vi "Format Fit Output.vi"(5 "Fit Model":T4, 7 "f(x,a)":T1, 8 "Error In":errorcluster, 9 "Fit Results":T2, 10 "Additional Data":variant, 11 "Data in":T3) -> (0 "Error Out":errorcluster, 1 "Fit Parameters Uncertainties Cluster":variant, 3 "Fit Parameters Cluster":variant)   [LabVIEW 2021, in "Fits.lvlib"]
uses:
  Fits.lvlib
  Fit Models.ctl
  <vilib>/gmath/NumericalOptimization/LM model function reference.ctl
  <vilib>/Utility/error.llb/DialogType.ctl
  Gaussian/Gaussian Fit Results v2.ctl
  Asymmetric Gaussian/Asymmetric Gaussian Fit Results v2.ctl
  Lorentzian/Lorentzian Fit Results v2.ctl
  Asymmetric Lorentzian/Asymmetric Lorentzian Fit Results v2.ctl
  Gaussian-Lorentzian/Gaussian-Lorentzian Fit Results v2.ctl
  Lorentzian-Gaussian/Lorentzian-Gaussian Fit Results v2.ctl
  D-Only Fixed Parameters.ctl
  Two Connected Gaussians/Two H-Connected Gaussians Fit Parameters.ctl
  Two Connected Gaussians/Two T-Connected Gaussians Fit Parameters.ctl
  Two Connected Asymmetric Gaussians/Two H-Connected Asymmetric Gaussians Fit Parameters.ctl
  Two Connected Asymmetric Gaussians/Two T-Connected Asymmetric Gaussians Fit Parameters.ctl
  Single Exponential/Single Exponential Fit Parameters v2.ctl
  Power Law/Power Law Fit Parameters.ctl
  IRF(X)PSED/IRF(X)PSED Fit Parameters.ctl
  IRF(X)PSED/IRF(X)PSED Fixed Parameters v3.ctl
  IRF(X)PSED/IRF(X)PSED Extraction Options.ctl
  IRF(X)PSED/Fourier Series Smoothing Option.ctl
  IRF(X)PSED/Fourier Series Truncation.ctl
  IRF(X)PSED/IRF Extraction Method.ctl
  Double Exponential/Double Exponential Fit Parameters v2.ctl
  ACF-CCF/2D ACF/2D Gaussian ACF Fit Results.ctl
  ACF-CCF/2D ACF/2D Gaussian + Blinking ACF Fit Results.ctl
  ACF-CCF/2D ACF/2D Gaussian + Flow ACF Fit Results.ctl
  ACF-CCF/3D ACF/3D Gaussian ACF Fit Results.ctl
  ACF-CCF/3D ACF/3D Gaussian + Blinking ACF Fit Results.ctl
  ACF-CCF/2D ACF/2D Gaussian ACF & 2D Gaussian ACF + Flow Fit Results.ctl
  <vilib>/Analysis/NI_AALPro.lvlib
  <vilib>/gmath/NI_Gmath.lvlib
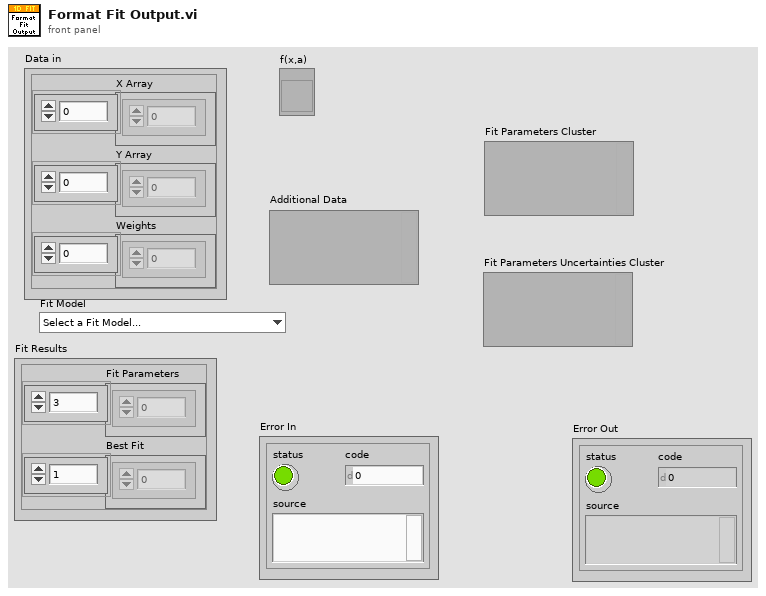
[diagram p1: front panel]
types:
  T1 = typedef "NI_Gmath.lvlib/LM model function reference.ctl" = refnum<vi>
  T2 = cluster{"Fit Parameters":dbl[], "Best Fit":dbl[]}
  T3 = cluster{"X Array":dbl[], "Y Array":dbl[], "Weights":dbl[]}
  T4 = typedef "Fits.lvlib/Fit Models.ctl" = enum16{"Select a Fit Model...", "           Single Peak", "Gaussian", "Asymmetric Gaussian", "Lorentzian", "Asymmetric Lorentzian", "Gaussian/Lorentzian", "Lorentzian/Gaussian", "           Double Peak", "Two Gaussians", "Two Asymmetric Gaussians", "Two H-Connected Gaussians", "Two T-Connected Gaussians", "Two H-Connected Asymmetric Gaussians", "Two T-Connected Asymmetric Gaussians", "           Triple Peak", "Three Gaussians", "Three Asymmetric Gaussians", "              Decays", "1-Exponential", "IRF*PSED", "2-Exponentials", "Power Law", "Power Law with Offset", "               ACF", "2D Gaussian ACF", "2D Gaussian + Blinking ACF", "2D Gaussian + Flow ACF", "3D Gaussian ACF", "3D Gaussian + Blinking ACF", "             Multiplot", "2D Gaussian ACF & 2D Gaussian + Flow ACF"}
  T5 = typedef "Fits.lvlib/D-Only Fixed Parameters.ctl" = cluster{"Fix D-only Peak Location":bool, "Peak Location":dbl, "Fix D-only Peak FWHM":bool, "Peak FWHM":dbl}
  T6 = typedef "Fits.lvlib/IRF(X)PSED Fixed Parameters v3.ctl" = cluster{"order":i32, "T":dbl, "Time Constant Array":dbl[], "{S_k, C_k, phi_k, e_k} arrays":cluster{"S_k Array":dbl[], "C_k Array":dbl[], "phi_k Array":dbl[], "e_k Array":dbl[]}, "IRF Extraction Options":T7}
  T7 = typedef "Fits.lvlib/IRF(X)PSED Extraction Options.ctl" = cluster{"Time Constant for IRF Extraction":dbl[unit], "IRF Order":i32, "Fourier Series Smoothing":T8, "Noise Threshold":dbl, "Smoothing Width":dbl, "Fourier Series Truncation":T9, "Truncation Order":i32, "Save Power Spectrum":bool, "Smoothing":bool, "Smoothing Parameter":dbl, "Smoothing Order":u32, "Method":T10}
  T8 = typedef "Fits.lvlib/Fourier Series Smoothing Option.ctl" = enum16{"None", "Lanczos Factors", "Fejer Summation"}
  T9 = typedef "Fits.lvlib/Fourier Series Truncation.ctl" = enum16{"Automatic", "Fixed"}
  T10 = typedef "Fits.lvlib/IRF Extraction Method.ctl" = enum16{"Direct", "Topless", "Toeplitz"}
  T11 = typedef "DialogType.ctl" = u16
  T12 = typedef "Fits.lvlib/Gaussian Fit Results v2.ctl" = cluster{"Amplitude":dbl, "Peak":dbl, "SDV":dbl, "FWHM":dbl, "Integral":dbl, "RMSE":dbl, "R^2":dbl}
  T13 = typedef "Fits.lvlib/Asymmetric Gaussian Fit Results v2.ctl" = cluster{"Amplitude":dbl, "Peak":dbl, "SDV-":dbl, "SDV+":dbl, "Mean":dbl, "SDV":dbl, "FWHM":dbl, "Integral":dbl, "RMSE":dbl, "R^2":dbl}
  T14 = typedef "Fits.lvlib/Lorentzian Fit Results v2.ctl" = cluster{"Amplitude":dbl, "Peak":dbl, "FWHM":dbl, "Integral":dbl, "RMSE":dbl, "R^2":dbl}
  T15 = typedef "Fits.lvlib/Asymmetric Lorentzian Fit Results v2.ctl" = cluster{"Amplitude":dbl, "Peak":dbl, "FWHM-":dbl, "FWHM+":dbl, "Integral":dbl, "RMSE":dbl, "R^2":dbl}
  T16 = typedef "Fits.lvlib/Gaussian-Lorentzian Fit Results v2.ctl" = cluster{"Amplitude":dbl, "Peak":dbl, "SDV-":dbl, "FWHM+":dbl, "Mean":dbl, "FWHM":dbl, "Integral":dbl, " RMSE":dbl, "R^2":dbl}
  T17 = typedef "Fits.lvlib/Lorentzian-Gaussian Fit Results v2.ctl" = cluster{"Amplitude":dbl, "Peak":dbl, "FWHM-":dbl, "SDV+":dbl, "Mean":dbl, "FWHM":dbl, "Integral":dbl, "RMSE":dbl, "R^2":dbl}
  T18 = typedef "Fits.lvlib/Two H-Connected Gaussians Fit Parameters.ctl" = cluster{"Gaussian Parameters":T12[], "Bridge Amplitude ":dbl}
  T19 = typedef "Fits.lvlib/Two T-Connected Gaussians Fit Parameters.ctl" = cluster{"Gaussian Parameters":T12[], "Bridge Amplitude ":dbl, "Bridge Slope":dbl}
  T20 = typedef "Fits.lvlib/Two H-Connected Asymmetric Gaussians Fit Parameters.ctl" = cluster{"Asymmetric Gaussian Parameters":T13[], "Bridge Amplitude":dbl}
  T21 = typedef "Fits.lvlib/Two T-Connected Asymmetric Gaussians Fit Parameters.ctl" = cluster{"Asymmetric Gaussian Parameters":T13[], "Bridge Amplitude":dbl, "Bridge Slope":dbl}
  T22 = typedef "Fits.lvlib/Single Exponential Fit Parameters v2.ctl" = cluster{"Amplitude":dbl, "Time Constant":dbl, "Baseline":dbl, "Mean":dbl, "SDV":dbl, "FWHM":dbl, "Integral":dbl, "MSE":dbl, "R^2":dbl}
  T23 = typedef "Fits.lvlib/Power Law Fit Parameters.ctl" = cluster{"A":dbl, "beta":dbl, "B":dbl, "Mean":dbl, "SDV":dbl, "Integral":dbl, "MSE":dbl, "R^2":dbl}
  T24 = typedef "Fits.lvlib/IRF(X)PSED Fit Parameters.ctl" = cluster{"Offset":dbl, "Amplitudes":dbl[], "Time Constants":dbl[], "Baseline":dbl, "Lifetime":dbl, "IRF order":dbl, "Period":dbl, "SDV":dbl, "FWHM":dbl, "Integral":dbl, "MSE":dbl, "R^2":dbl}
  T25 = typedef "Fits.lvlib/Double Exponential Fit Parameters v2.ctl" = cluster{"A1":dbl, "tau1":dbl, "A2":dbl, "tau2":dbl, "Baseline":dbl, "Mean":dbl, "SDV":dbl, "Integral":dbl, "MSE":dbl, "R^2":dbl}
  T26 = typedef "Fits.lvlib/2D Gaussian ACF Fit Results.ctl" = cluster{"Amplitude":dbl, "Diffusion Time":dbl, "RMSE":dbl, "R^2":dbl}
  T27 = typedef "Fits.lvlib/2D Gaussian + Blinking ACF Fit Results.ctl" = cluster{"Amplitude":dbl, "Diffusion Time":dbl, "Blinking Fraction":dbl, "Blinking Time Constant":dbl, "RMSE":dbl, "R^2":dbl}
  T28 = typedef "Fits.lvlib/2D Gaussian + Flow ACF Fit Results.ctl" = cluster{"Amplitude":dbl, "Diffusion Time":dbl, "Translation Time":dbl, "RMSE":dbl, "R^2":dbl}
  T29 = typedef "Fits.lvlib/3D Gaussian ACF Fit Results.ctl" = cluster{"Amplitude":dbl, "Diffusion Time":dbl, "Aspect Ratio":dbl, "RMSE":dbl, "R^2":dbl}
  T30 = typedef "Fits.lvlib/3D Gaussian + Blinking ACF Fit Results.ctl" = cluster{"Amplitude":dbl, "Diffusion Time":dbl, "Aspect Ratio":dbl, "Blinking Fraction":dbl, "Blinking Time Constant":dbl, "RMSE":dbl, "R^2":dbl}
  T31 = typedef "Fits.lvlib/2D Gaussian ACF & 2D Gaussian ACF + Flow Fit Results.ctl" = cluster{"Amplitude 1":dbl, "Diffusion Time":dbl, "Amplitude 2":dbl, "Translation Time":dbl, "RMSE":dbl, "R^2":dbl}
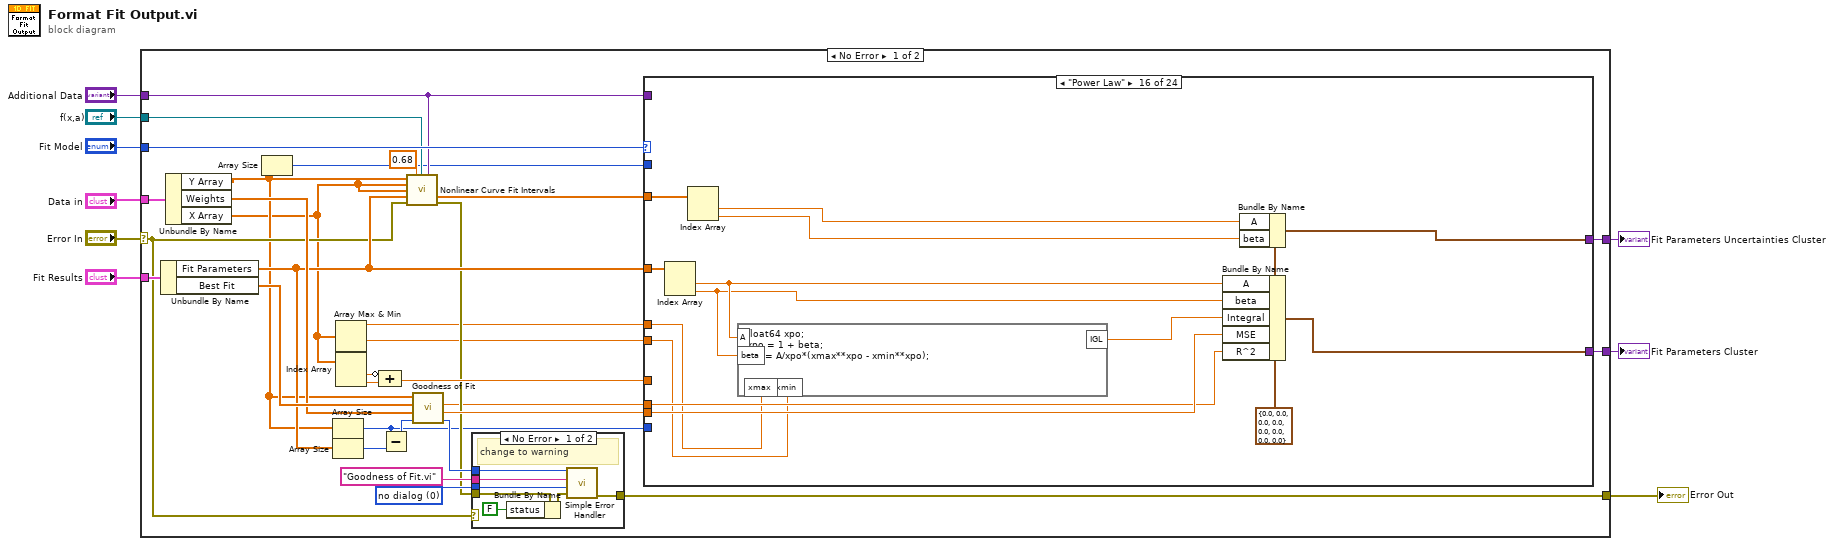
[diagram p0: block diagram]
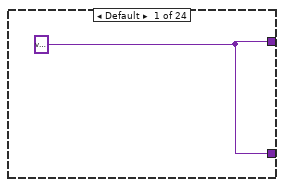
[diagram p3: hidden frame]
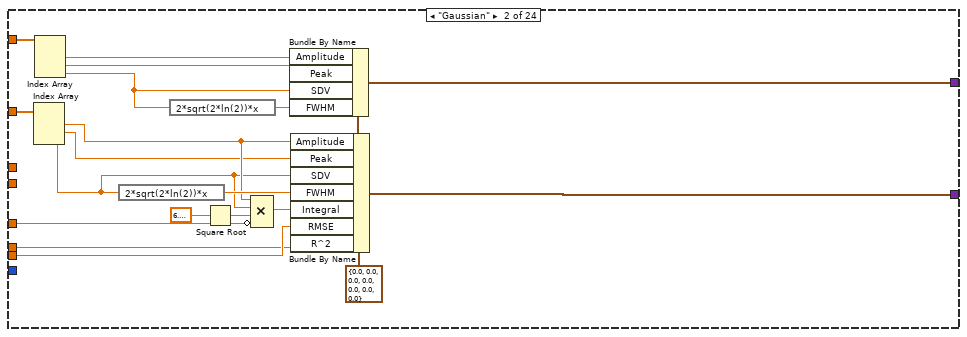
[diagram p4: hidden frame]
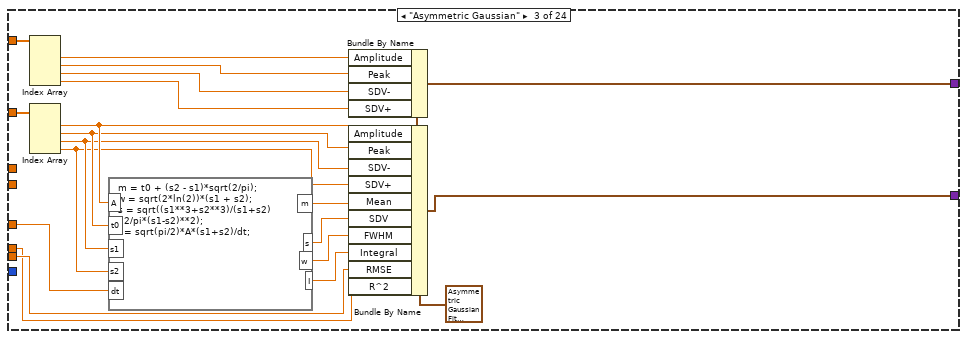
[diagram p5: hidden frame]
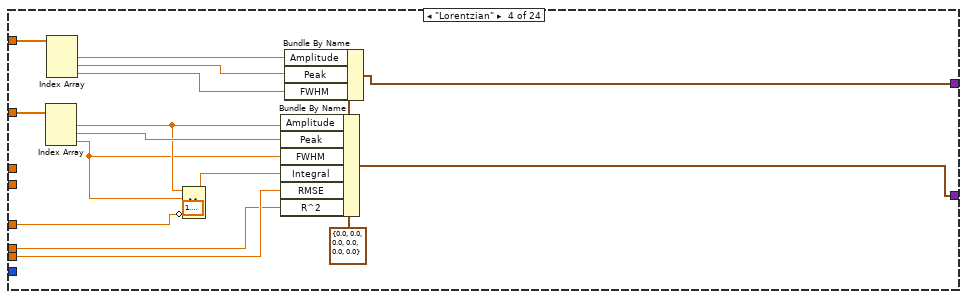
[diagram p6: hidden frame]
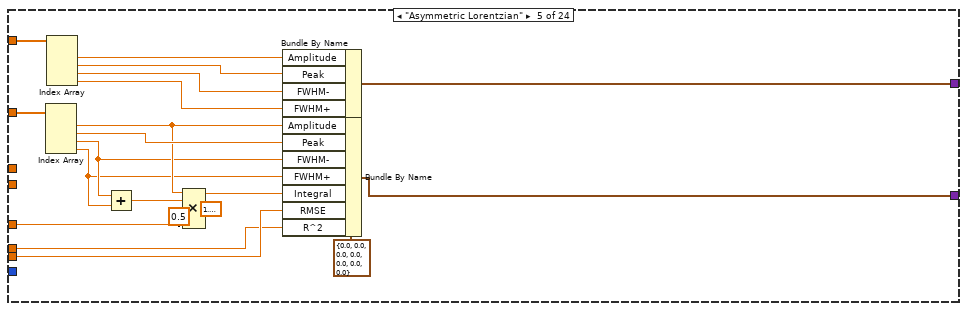
[diagram p7: hidden frame]
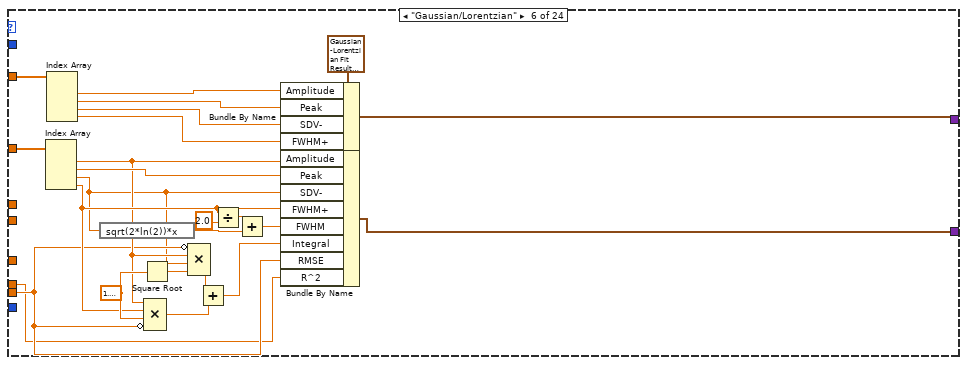
[diagram p8: hidden frame]
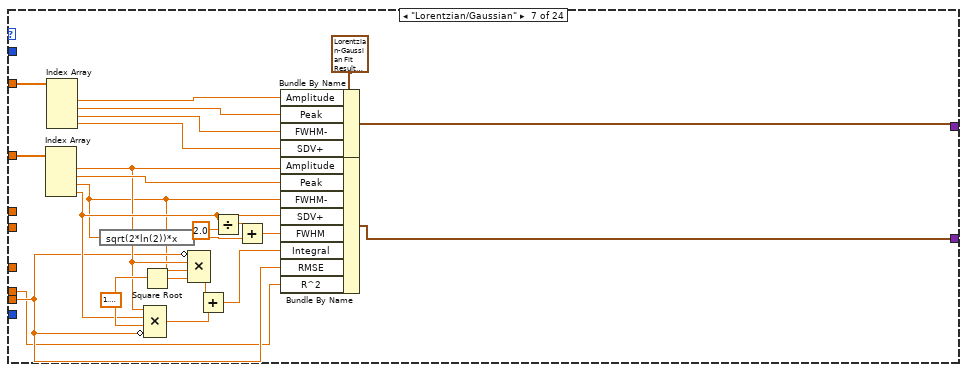
[diagram p9: hidden frame]
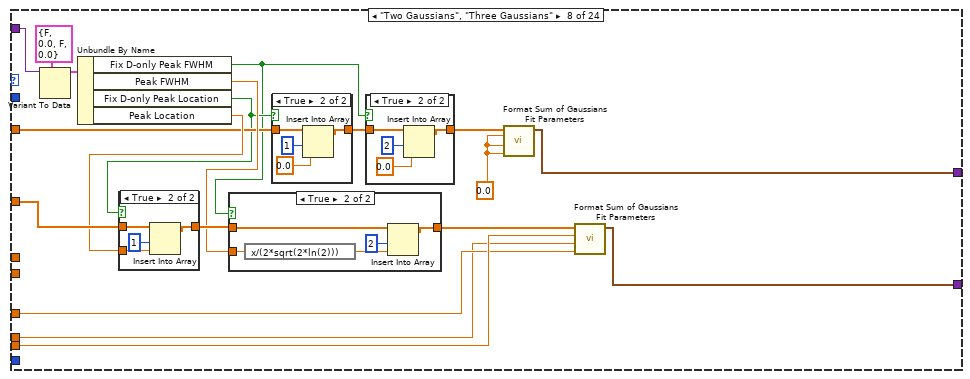
[diagram p10: hidden frame]
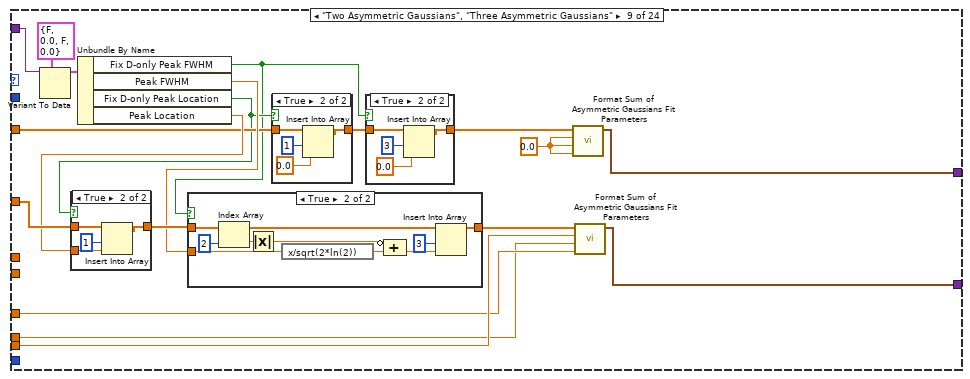
[diagram p15: hidden frame]
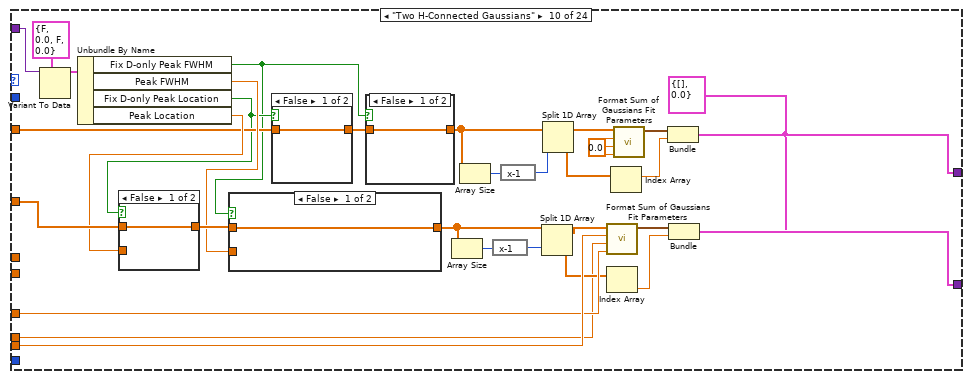
[diagram p20: hidden frame]
diagram:
  n1 = case shown="No Error" "Error In" {
    selector: "Error In" -> [w15 w667]
    tunnel: [w40 _] -> w9
    tunnel: [w39 _] -> w8
    tunnel: "Data in" -> [w32 _]
    tunnel: "Fit Results" -> [w31 _]
    tunnel: "Fit Model" -> [w29 _]
    tunnel: "f(x,a)" -> [w25 _]
    tunnel: [w20 w667] -> w2
    tunnel: "Additional Data" -> [w18 _]
    frame No Error {
      w22 = T11 0 items=["no dialog", "OK message", "continue or stop message", "OK message + warnings", "continue/stop + warnings"] ("type of dialog (OK msg:1)")
      n2 = Unbundle By Name(w31) -> ("Fit Parameters"=w27:dbl[], "Best Fit"=w30:dbl[])
      n3 = Unbundle By Name(w32) -> ("Y Array"=w14:dbl[], "Weights"=w28:dbl[], "X Array"=w12:dbl[])
      n4 = Array Size(array=w14) -> (size(s)=w13:i32)
      n5 = Array Size(array=w14) -> (size(s)=w16:i32)
      n6 = Array Size(array=w27) -> (size(s)=w35:i32)
      n7 = Array Max & Min(array=w12) -> (max value=w10:dbl, min value=w11:dbl)  [unwired: 2 out]
      n8 = Index Array(array=w12) -> (element #1=w36:dbl, element #2=w38:dbl)  [unwired: 2 in]
      n9 = Compound Arithmetic op=ADD(invert w36, w38) -> (w37:dbl)
      n10 = Subtract(x=w16, y=w35) -> (x-y=w34:i32)
      n11 = call <vilib>:"Nonlinear Curve Fit Intervals.vi"("Y"=w14, "confidence level"=0.68, "f(x,a)"=w25, "data"=w18, "X"=w12, "Weight"=w12, "best fit parameters"=w27, "error in (no error)"=w15) -> ("delta best fit parameters"=w26:dbl[], "error out"=w21:errorcluster)  [unwired: 4 in, 2 out]
      n12 = call <vilib>:"Goodness of Fit.vi"("degree of freedom"=w34, "Weight"=w28, "Best Fit"=w30, "Y"=w14) -> ("error"=w24:i32, "RMSE"=w33:dbl, "R-square"=w17:dbl)  [unwired: 4 in, 1 out]
      n13 = case shown="No Error" w15 {
        selector: w15 -> [_ w48]
        tunnel: w24 -> [w47 _]
        tunnel: "Goodness of Fit.vi" ("error source (\" \")") -> [w46 _]
        tunnel: w22 -> [w45 _]
        tunnel: w21 -> [w44 _]
        tunnel: [w43 w48] -> w20
        frame No Error {
          # "change to warning"
          n14 = Bundle By Name(cluster=w44, "status"=FALSE) -> (w42:errorcluster)
          n15 = call <vilib>:"Simple Error Handler.vi"("error code (no error:0)"=w47, "error source (\" \")"=w46, "type of dialog (OK msg:1)"=w45, "error in (no error)"=w42) -> ("error out"=w43:errorcluster)  [unwired: 1 in, 4 out]
        }
        frame Error {
        }
      }
      n16 = case shown="\"Power Law\"" w29 {
        tunnel: [w49 w56 w82 w90 w114 w142 w166 w176 w216 w274 w329 w382 w441 w489 w510 w524 w557 w576 w589 w604 w617 w632 w649 w664] -> w40
        tunnel: [w49 w55 w81 w102 w113 w141 w165 w175 w215 w275 w330 w383 w442 w488 w509 w523 w556 w568 w588 w603 w616 w631 w648 w663] -> w39
        tunnel: w37 -> [_ w59 w71 w97 w119 _ _ w178 w218 w276 w331 w384 w443 w483 _ _ w554 w574 _ _ _ _ _ _]
        tunnel: w33 -> [_ w58 w80 w103 w123 w127 w152 w179 w219 w277 w332 w385 w444 w492 w511 w525 w558 w570 w591 w606 w619 w634 w651 w666]
        tunnel: w27 -> [_ w57 w88 w104 w124 w148 w172 w188 w228 w285 w340 w393 w452 w496 w512 w526 w547 w575 w590 w605 w618 w633 w650 w665]
        tunnel: w26 -> [_ w54 w87 w95 w118 w146 w170 w184 w224 w281 w336 w389 w448 w499 w515 w529 w552 w581 w587 w602 w615 w630 w647 w662]
        tunnel: w18 -> [_ _ _ _ _ _ _ w190 w230 w287 w342 w395 w454 _ _ _ w541 _ _ _ _ _ _ _]
        tunnel: w17 -> [_ w50 w69 w89 w105 w125 w149 w174 w213 w258 w310 w365 w423 w486 w507 w522 w555 w563 w585 w600 w613 w629 w645 w660]
        tunnel: w16 -> [_ _ _ _ _ _ _ _ _ _ _ _ _ w482 _ _ w553 w561 _ _ _ _ _ _]
        tunnel: w13 -> [_ _ _ _ _ _ _ _ _ _ _ _ _ _ _ _ w532 _ _ _ _ _ _ _]
        tunnel: w11 -> [_ _ _ _ _ _ _ _ _ _ _ _ _ _ w502 w518 _ _ _ _ _ _ _ _]
        tunnel: w10 -> [_ _ _ _ _ _ _ _ _ _ _ _ _ _ w501 w517 _ _ _ _ _ _ _ _]
        frame Default {
          w49 = variant
        }
        frame "Gaussian" {
          w67 = T12 {"Amplitude"=0.0, "Peak"=0.0, "SDV"=0.0, "FWHM"=0.0, "Integral"=0.0, "RMSE"=0.0, "R^2"=0.0} ("Gaussian Fit Parameters")
          n17 = Index Array(array=w57) -> (element #1=w62:dbl, element #2=w61:dbl, element #3=w60:dbl)  [unwired: 3 in]
          n18 = Index Array(array=w54) -> (element #1=w53:dbl, element #2=w52:dbl, element #3=w51:dbl)  [unwired: 3 in]
          n19 = expression code="2*sqrt(2*ln(2))*x"(w60) -> (w66:dbl)
          n20 = expression code="2*sqrt(2*ln(2))*x"(w51) -> (w68:dbl)
          n21 = Square Root(x=6.283185307179586) -> (sqrt(x)=w64:dbl)
          n22 = Compound Arithmetic op=MULTIPLY(w62, w60, w64, invert w59) -> (w65:dbl)
          n23 = Bundle By Name(cluster=w67, "Amplitude"=w53, "Peak"=w52, "SDV"=w51, "FWHM"=w68) -> (w56:T12)
          n24 = Bundle By Name(cluster=w67, "Amplitude"=w62, "Peak"=w61, "SDV"=w60, "FWHM"=w66, "Integral"=w65, "RMSE"=w58, "R^2"=w50) -> (w55:T12)
        }
        frame "Asymmetric Gaussian" {
          w86 = T13 {"Amplitude"=0.0, "Peak"=0.0, "SDV-"=0.0, "SDV+"=0.0, "Mean"=0.0, "SDV"=0.0, "FWHM"=0.0, "Integral"=0.0, "RMSE"=0.0, "R^2"=0.0} ("Lorentz Fit Parameters")
          n25 = Index Array(array=w87) -> (element #1=w85:dbl, element #2=w84:dbl, element #3=w83:dbl, element #4=w70:dbl)  [unwired: 4 in]
          n26 = Index Array(array=w88) -> (element #1=w75:dbl, element #2=w74:dbl, element #3=w73:dbl, element #4=w72:dbl)  [unwired: 4 in]
          n27 = formula code="m = t0 + (s2 - s1)*sqrt(2/pi);\nw = sqrt(2*ln(2))*(s1 + s2);\ns = sqrt((s1**3+s2**3)/(s1+s2)\n- 2/pi*(s1-s2)**2);\nI = sqrt(pi/2)*A*(s1+s2)/dt;"("t0"=w74, "s1"=w73, "s2"=w72, "A"=w75, "dt"=w71) -> ("m"=w76:dbl, "w"=w78:dbl, "s"=w77:dbl, "I"=w79:dbl)
          n28 = Bundle By Name(cluster=w86, "Amplitude"=w85, "Peak"=w84, "SDV-"=w83, "SDV+"=w70) -> (w82:T13)
          n29 = Bundle By Name(cluster=w86, "Amplitude"=w75, "Peak"=w74, "SDV-"=w73, "SDV+"=w72, "Mean"=w76, "SDV"=w77, "FWHM"=w78, "Integral"=w79, "RMSE"=w80, "R^2"=w69) -> (w81:T13)
        }
        frame "Lorentzian" {
          w94 = T14 {"Amplitude"=0.0, "Peak"=0.0, "FWHM"=0.0, "Integral"=0.0, "RMSE"=0.0, "R^2"=0.0} ("Lorentz Fit Parameters")
          n30 = Index Array(array=w104) -> (element #1=w100:dbl, element #2=w101:dbl, element #3=w99:dbl)  [unwired: 3 in]
          n31 = Index Array(array=w95) -> (element #1=w93:dbl, element #2=w92:dbl, element #3=w91:dbl)  [unwired: 3 in]
          n32 = Compound Arithmetic op=MULTIPLY(w100, w99, 1.5707963267948966, invert w97) -> (w96:dbl)
          n33 = Bundle By Name(cluster=w94, "Amplitude"=w100, "Peak"=w101, "FWHM"=w99, "Integral"=w96, "RMSE"=w103, "R^2"=w89) -> (w102:T14)
          n34 = Bundle By Name(cluster=w94, "Amplitude"=w93, "Peak"=w92, "FWHM"=w91) -> (w90:T14)
        }
        frame "Asymmetric Lorentzian" {
          w112 = T15 {"Amplitude"=0.0, "Peak"=0.0, "FWHM-"=0.0, "FWHM+"=0.0, "Integral"=0.0, "RMSE"=0.0, "R^2"=0.0} ("Asymmetric Lorentz Fit Parameters")
          n35 = Index Array(array=w124) -> (element #1=w121:dbl, element #2=w122:dbl, element #3=w110:dbl, element #4=w109:dbl)  [unwired: 4 in]
          n36 = Index Array(array=w118) -> (element #1=w117:dbl, element #2=w116:dbl, element #3=w115:dbl, element #4=w111:dbl)  [unwired: 4 in]
          n37 = Add(x=w110, y=w109) -> (x+y=w108:dbl)
          n38 = Compound Arithmetic op=MULTIPLY(w121, w108, 1.5707963267948966, 0.5 ("value"), invert w119) -> (w106:dbl)
          n39 = Bundle By Name(cluster=w112, "Amplitude"=w117, "Peak"=w116, "FWHM-"=w115, "FWHM+"=w111) -> (w114:T15)
          n40 = Bundle By Name(cluster=w112, "Amplitude"=w121, "Peak"=w122, "FWHM-"=w110, "FWHM+"=w109, "Integral"=w106, "RMSE"=w123, "R^2"=w105) -> (w113:T15)
        }
        frame "Gaussian/Lorentzian" {
          w137 = 1.5707963267948966
          w140 = T16 {"Amplitude"=0.0, "Peak"=0.0, "SDV-"=0.0, "FWHM+"=0.0, "Mean"=0.0, "FWHM"=0.0, "Integral"=0.0, " RMSE"=0.0, "R^2"=0.0} ("Gaussian/Lorentzian Fit Parameters")
          n41 = Index Array(array=w148) -> (element #1=w128:dbl, element #2=w147:dbl, element #3=w126:dbl, element #4=w129:dbl)  [unwired: 4 in]
          n42 = Index Array(array=w146) -> (element #1=w145:dbl, element #2=w144:dbl, element #3=w143:dbl, element #4=w139:dbl)  [unwired: 4 in]
          n43 = expression code="sqrt(2*ln(2))*x"(w126) -> (w132:dbl)
          n44 = Square Root(x=w137) -> (sqrt(x)=w138:dbl)
          n45 = Compound Arithmetic op=MULTIPLY(w128, w129, w137, invert w127) -> (w136:dbl)
          n46 = Compound Arithmetic op=MULTIPLY(invert w127, w128, w126, w138) -> (w135:dbl)
          n47 = Add(x=w135, y=w136) -> (x+y=w130:dbl)
          n48 = Divide(x=w129, y=2.0) -> (x/y=w134:dbl)
          n49 = Add(x=w134, y=w132) -> (x+y=w131:dbl)
          n50 = Bundle By Name(cluster=w140, "Amplitude"=w145, "Peak"=w144, "SDV-"=w143, "FWHM+"=w139) -> (w142:T16)
          n51 = Bundle By Name(cluster=w140, "Amplitude"=w128, "Peak"=w147, "SDV-"=w126, "FWHM+"=w129, "FWHM"=w131, "Integral"=w130, "RMSE"=w127, "R^2"=w125) -> (w141:T16)
        }
        frame "Lorentzian/Gaussian" {
          w150 = T17 {"Amplitude"=0.0, "Peak"=0.0, "FWHM-"=0.0, "SDV+"=0.0, "Mean"=0.0, "FWHM"=0.0, "Integral"=0.0, "RMSE"=0.0, "R^2"=0.0} ("Lorentzian/Gaussian Fit Parameters")
          w162 = 1.5707963267948966
          n52 = Index Array(array=w172) -> (element #1=w153:dbl, element #2=w171:dbl, element #3=w151:dbl, element #4=w154:dbl)  [unwired: 4 in]
          n53 = Index Array(array=w170) -> (element #1=w169:dbl, element #2=w168:dbl, element #3=w167:dbl, element #4=w164:dbl)  [unwired: 4 in]
          n54 = expression code="sqrt(2*ln(2))*x"(w151) -> (w157:dbl)
          n55 = Square Root(x=w162) -> (sqrt(x)=w163:dbl)
          n56 = Compound Arithmetic op=MULTIPLY(w153, w154, w162, invert w152) -> (w161:dbl)
          n57 = Compound Arithmetic op=MULTIPLY(invert w152, w153, w151, w163) -> (w160:dbl)
          n58 = Add(x=w160, y=w161) -> (x+y=w155:dbl)
          n59 = Divide(x=w154, y=2.0) -> (x/y=w159:dbl)
          n60 = Add(x=w159, y=w157) -> (x+y=w156:dbl)
          n61 = Bundle By Name(cluster=w150, "Amplitude"=w169, "Peak"=w168, "FWHM-"=w167, "SDV+"=w164) -> (w166:T17)
          n62 = Bundle By Name(cluster=w150, "Amplitude"=w153, "Peak"=w171, "FWHM-"=w151, "SDV+"=w154, "FWHM"=w156, "Integral"=w155, "RMSE"=w152, "R^2"=w149) -> (w165:T17)
        }
        frame "Two Gaussians", "Three Gaussians" {
          w173 = 0.0 ("MSE")
          n63 = Variant To Data(type=T5 {"Fix D-only Peak Location"=FALSE, "Peak Location"=0.0, "Fix D-only Peak FWHM"=FALSE, "Peak FWHM"=0.0} ("Fixed Parameters"), Variant=w190) -> (data=w189:T5)  [unwired: 1 in, 1 out]
          n64 = Unbundle By Name(w189) -> ("Fix D-only Peak FWHM"=w181:bool, "Peak FWHM"=w185:dbl, "Fix D-only Peak Location"=w183:bool, "Peak Location"=w186:dbl)
          n65 = case shown="True" w183 {
            tunnel: w188 -> [w208 w212]
            tunnel: [w208 w211] -> w187
            tunnel: w186 -> [_ w209]
            frame False {
            }
            frame True {
              n66 = Insert Into Array(array=w212, index=1 ("length"), new element=w209) -> (w211:dbl[])
            }
          }
          n67 = case shown="True" w181 {
            tunnel: w187 -> [w202 w207]
            tunnel: [w202 w206] -> w180
            tunnel: w185 -> [_ w204]
            frame False {
            }
            frame True {
              n68 = expression code="x/(2*sqrt(2*ln(2)))"(w204) -> (w203:dbl)
              n69 = Insert Into Array(array=w207, index=2, new element=w203) -> (w206:dbl[])
            }
          }
          n70 = case shown="True" w183 {
            tunnel: w184 -> [w197 w201]
            tunnel: [w197 w200] -> w182
            frame False {
            }
            frame True {
              n71 = Insert Into Array(array=w201, index=1 ("length"), new element=0.0 ("new element/subarray")) -> (w200:dbl[])
            }
          }
          n72 = case shown="True" w181 {
            tunnel: w182 -> [w192 w196]
            tunnel: [w192 w195] -> w177
            frame False {
            }
            frame True {
              n73 = Insert Into Array(array=w196, index=2, new element=0.0 ("new element/subarray")) -> (w195:dbl[])
            }
          }
          n74 = call "Format Sum of Gaussians Fit Parameters.vi"("Step Size"=w173, "R^2"=w173, "MSE"=w173, "Best Fit Parameters"=w177) -> ("Array of Gaussian Fit Parameters"=w176:T12[])  [unwired: 6 in, 1 out]
          n75 = call "Format Sum of Gaussians Fit Parameters.vi"("Step Size"=w178, "R^2"=w174, "MSE"=w179, "Best Fit Parameters"=w180) -> ("Array of Gaussian Fit Parameters"=w175:T12[])  [unwired: 6 in, 1 out]
        }
        frame "Two Asymmetric Gaussians", "Three Asymmetric Gaussians" {
          w214 = 0.0 ("MSE")
          n76 = Variant To Data(type=T5 {"Fix D-only Peak Location"=FALSE, "Peak Location"=0.0, "Fix D-only Peak FWHM"=FALSE, "Peak FWHM"=0.0} ("Fixed Parameters"), Variant=w230) -> (data=w229:T5)  [unwired: 1 in, 1 out]
          n77 = Unbundle By Name(w229) -> ("Fix D-only Peak FWHM"=w221:bool, "Peak FWHM"=w225:dbl, "Fix D-only Peak Location"=w223:bool, "Peak Location"=w226:dbl)
          n78 = case shown="True" w223 {
            tunnel: w228 -> [w252 w256]
            tunnel: [w252 w255] -> w227
            tunnel: w226 -> [_ w253]
            frame False {
            }
            frame True {
              n79 = Insert Into Array(array=w256, index=1 ("length"), new element=w253) -> (w255:dbl[])
            }
          }
          n80 = case shown="True" w221 {
            tunnel: w227 -> [w242 w247]
            tunnel: [w242 w251] -> w220
            tunnel: w225 -> [_ w249]
            frame False {
            }
            frame True {
              n81 = Index Array(array=w247, index=2) -> (element=w244:dbl)
              n82 = Absolute Value(x=w244) -> (abs(x)=w243:dbl)
              n83 = expression code="x/sqrt(2*ln(2))"(w249) -> (w248:dbl)
              n84 = Compound Arithmetic op=ADD(invert w243, w248) -> (w245:dbl)
              n85 = Insert Into Array(array=w247, index=3, new element=w245) -> (w251:dbl[])
            }
          }
          n86 = case shown="True" w223 {
            tunnel: w224 -> [w237 w241]
            tunnel: [w237 w240] -> w222
            frame False {
            }
            frame True {
              n87 = Insert Into Array(array=w241, index=1 ("length"), new element=0.0 ("new element/subarray")) -> (w240:dbl[])
            }
          }
          n88 = case shown="True" w221 {
            tunnel: w222 -> [w232 w236]
            tunnel: [w232 w235] -> w217
            frame False {
            }
            frame True {
              n89 = Insert Into Array(array=w236, index=3, new element=0.0 ("new element/subarray")) -> (w235:dbl[])
            }
          }
          n90 = call "Format Sum of Asymmetric Gaussians Fit Parameters.vi"("Step Size"=w214, "R^2"=w214, "MSE"=w214, "Best Fit Parameters"=w217) -> ("Array of Asymmetric Gaussian Fit Parameters"=w216:T13[])  [unwired: 6 in, 1 out]
          n91 = call "Format Sum of Asymmetric Gaussians Fit Parameters.vi"("Step Size"=w218, "R^2"=w213, "MSE"=w219, "Best Fit Parameters"=w220) -> ("Array of Asymmetric Gaussian Fit Parameters"=w215:T13[])  [unwired: 6 in, 1 out]
        }
        frame "Two H-Connected Gaussians" {
          w261 = T18 {"Gaussian Parameters"=[], "Bridge Amplitude "=0.0} ("Bridged Gaussians Parameters")
          w257 = 0.0 ("MSE")
          n92 = Variant To Data(type=T5 {"Fix D-only Peak Location"=FALSE, "Peak Location"=0.0, "Fix D-only Peak FWHM"=FALSE, "Peak FWHM"=0.0} ("Fixed Parameters"), Variant=w287) -> (data=w286:T5)  [unwired: 1 in, 1 out]
          n93 = Unbundle By Name(w286) -> ("Fix D-only Peak FWHM"=w278:bool, "Peak FWHM"=w282:dbl, "Fix D-only Peak Location"=w280:bool, "Peak Location"=w283:dbl)
          n94 = case shown="False" w280 {
            tunnel: w285 -> [w305 w309]
            tunnel: [w305 w308] -> w284
            tunnel: w283 -> [_ w306]
            frame False {
            }
            frame True {
              n95 = Insert Into Array(array=w309, index=1 ("length"), new element=w306) -> (w308:dbl[])
            }
          }
          n96 = case shown="False" w278 {
            tunnel: w284 -> [w299 w304]
            tunnel: [w299 w303] -> w268
            tunnel: w282 -> [_ w301]
            frame False {
            }
            frame True {
              n97 = expression code="x/(2*sqrt(2*ln(2)))"(w301) -> (w300:dbl)
              n98 = Insert Into Array(array=w304, index=2, new element=w300) -> (w303:dbl[])
            }
          }
          n99 = case shown="False" w280 {
            tunnel: w281 -> [w294 w298]
            tunnel: [w294 w297] -> w279
            frame False {
            }
            frame True {
              n100 = Insert Into Array(array=w298, index=1 ("length"), new element=0.0 ("new element/subarray")) -> (w297:dbl[])
            }
          }
          n101 = case shown="False" w278 {
            tunnel: w279 -> [w289 w293]
            tunnel: [w289 w292] -> w272
            frame False {
            }
            frame True {
              n102 = Insert Into Array(array=w293, index=2, new element=0.0 ("new element/subarray")) -> (w292:dbl[])
            }
          }
          n103 = Array Size(array=w268) -> (size(s)=w269:i32)
          n104 = Array Size(array=w272) -> (size(s)=w271:i32)
          n105 = expression code="x-1"(w269) -> (w267:i32)
          n106 = expression code="x-1"(w271) -> (w270:i32)
          n107 = Split 1D Array(array=w268, index=w267) -> (first subarray=w266:dbl[], second subarray=w260:dbl[])
          n108 = Split 1D Array(array=w272, index=w270) -> (first subarray=w273:dbl[], second subarray=w264:dbl[])
          n109 = call "Format Sum of Gaussians Fit Parameters.vi"("Step Size"=w276, "R^2"=w258, "MSE"=w277, "Best Fit Parameters"=w266) -> ("Array of Gaussian Fit Parameters"=w262:T12[])  [unwired: 6 in, 1 out]
          n110 = Index Array(array=w260) -> (element=w259:dbl)  [unwired: 1 in]
          n111 = Index Array(array=w264) -> (element=w263:dbl)  [unwired: 1 in]
          n112 = call "Format Sum of Gaussians Fit Parameters.vi"("Step Size"=w257, "R^2"=w257, "MSE"=w257, "Best Fit Parameters"=w273) -> ("Array of Gaussian Fit Parameters"=w265:T12[])  [unwired: 6 in, 1 out]
          n113 = Bundle(cluster=w261, "Gaussian Parameters"=w265, "Bridge Amplitude"=w263) -> (w274:T18)
          n114 = Bundle(cluster=w261, "Gaussian Parameters"=w262, "Bridge Amplitude"=w259) -> (w275:T18)
        }
        frame "Two T-Connected Gaussians" {
          w316 = T19 {"Gaussian Parameters"=[], "Bridge Amplitude "=0.0, "Bridge Slope"=0.0} ("Bridged Gaussians Parameters")
          w311 = 0.0 ("MSE")
          n115 = Variant To Data(type=T5 {"Fix D-only Peak Location"=FALSE, "Peak Location"=0.0, "Fix D-only Peak FWHM"=FALSE, "Peak FWHM"=0.0} ("Fixed Parameters"), Variant=w342) -> (data=w341:T5)  [unwired: 1 in, 1 out]
          n116 = Unbundle By Name(w341) -> ("Fix D-only Peak FWHM"=w333:bool, "Peak FWHM"=w337:dbl, "Fix D-only Peak Location"=w335:bool, "Peak Location"=w338:dbl)
          n117 = case shown="True" w335 {
            tunnel: w340 -> [w360 w364]
            tunnel: [w360 w363] -> w339
            tunnel: w338 -> [_ w361]
            frame False {
            }
            frame True {
              n118 = Insert Into Array(array=w364, index=1 ("length"), new element=w361) -> (w363:dbl[])
            }
          }
          n119 = case shown="True" w333 {
            tunnel: w339 -> [w354 w359]
            tunnel: [w354 w358] -> w323
            tunnel: w337 -> [_ w356]
            frame False {
            }
            frame True {
              n120 = expression code="x/(2*sqrt(2*ln(2)))"(w356) -> (w355:dbl)
              n121 = Insert Into Array(array=w359, index=2, new element=w355) -> (w358:dbl[])
            }
          }
          n122 = case shown="True" w335 {
            tunnel: w336 -> [w349 w353]
            tunnel: [w349 w352] -> w334
            frame False {
            }
            frame True {
              n123 = Insert Into Array(array=w353, index=1 ("length"), new element=0.0 ("new element/subarray")) -> (w352:dbl[])
            }
          }
          n124 = case shown="True" w333 {
            tunnel: w334 -> [w344 w348]
            tunnel: [w344 w347] -> w327
            frame False {
            }
            frame True {
              n125 = Insert Into Array(array=w348, index=2, new element=0.0 ("new element/subarray")) -> (w347:dbl[])
            }
          }
          n126 = Array Size(array=w323) -> (size(s)=w324:i32)
          n127 = Array Size(array=w327) -> (size(s)=w326:i32)
          n128 = expression code="x-2"(w324) -> (w322:i32)
          n129 = expression code="x-2"(w326) -> (w325:i32)
          n130 = Split 1D Array(array=w323, index=w322) -> (first subarray=w321:dbl[], second subarray=w315:dbl[])
          n131 = Split 1D Array(array=w327, index=w325) -> (first subarray=w328:dbl[], second subarray=w319:dbl[])
          n132 = call "Format Sum of Gaussians Fit Parameters.vi"("Step Size"=w331, "R^2"=w310, "MSE"=w332, "Best Fit Parameters"=w321) -> ("Array of Gaussian Fit Parameters"=w317:T12[])  [unwired: 6 in, 1 out]
          n133 = Index Array(array=w315) -> (element #1=w314:dbl, element #2=w312:dbl)  [unwired: 2 in]
          n134 = Index Array(array=w319) -> (element #1=w318:dbl, element #2=w313:dbl)  [unwired: 2 in]
          n135 = call "Format Sum of Gaussians Fit Parameters.vi"("Step Size"=w311, "R^2"=w311, "MSE"=w311, "Best Fit Parameters"=w328) -> ("Array of Gaussian Fit Parameters"=w320:T12[])  [unwired: 6 in, 1 out]
          n136 = Bundle By Name(cluster=w316, "Gaussian Parameters"=w320, "Bridge Amplitude"=w318, "Bridge Slope"=w313) -> (w329:T19)
          n137 = Bundle By Name(cluster=w316, "Gaussian Parameters"=w317, "Bridge Amplitude"=w314, "Bridge Slope"=w312) -> (w330:T19)
        }
        frame "Two H-Connected Asymmetric Gaussians" {
          w373 = T20 {"Asymmetric Gaussian Parameters"=[], "Bridge Amplitude"=0.0} ("output cluster")
          w366 = 0.0 ("MSE")
          n138 = Variant To Data(type=T5 {"Fix D-only Peak Location"=FALSE, "Peak Location"=0.0, "Fix D-only Peak FWHM"=FALSE, "Peak FWHM"=0.0} ("Fixed Parameters"), Variant=w395) -> (data=w394:T5)  [unwired: 1 in, 1 out]
          n139 = Unbundle By Name(w394) -> ("Fix D-only Peak FWHM"=w386:bool, "Peak FWHM"=w390:dbl, "Fix D-only Peak Location"=w388:bool, "Peak Location"=w391:dbl)
          n140 = case shown="True" w388 {
            tunnel: w393 -> [w417 w421]
            tunnel: [w417 w420] -> w392
            tunnel: w391 -> [_ w418]
            frame False {
            }
            frame True {
              n141 = Insert Into Array(array=w421, index=1 ("length"), new element=w418) -> (w420:dbl[])
            }
          }
          n142 = case shown="True" w386 {
            tunnel: w392 -> [w407 w412]
            tunnel: [w407 w416] -> w369
            tunnel: w390 -> [_ w414]
            frame False {
            }
            frame True {
              n143 = Index Array(array=w412, index=2) -> (element=w409:dbl)
              n144 = Absolute Value(x=w409) -> (abs(x)=w408:dbl)
              n145 = expression code="x/sqrt(2*ln(2))"(w414) -> (w413:dbl)
              n146 = Compound Arithmetic op=ADD(invert w408, w413) -> (w410:dbl)
              n147 = Insert Into Array(array=w412, index=3, new element=w410) -> (w416:dbl[])
            }
          }
          n148 = case shown="True" w388 {
            tunnel: w389 -> [w402 w406]
            tunnel: [w402 w405] -> w387
            frame False {
            }
            frame True {
              n149 = Insert Into Array(array=w406, index=1 ("length"), new element=0.0 ("new element/subarray")) -> (w405:dbl[])
            }
          }
          n150 = case shown="True" w386 {
            tunnel: w387 -> [w397 w401]
            tunnel: [w397 w400] -> w379
            frame False {
            }
            frame True {
              n151 = Insert Into Array(array=w401, index=3, new element=0.0 ("new element/subarray")) -> (w400:dbl[])
            }
          }
          n152 = Array Size(array=w379) -> (size(s)=w381:i32)
          n153 = Array Size(array=w369) -> (size(s)=w371:i32)
          n154 = expression code="x-1"(w381) -> (w380:i32)
          n155 = expression code="x-1"(w371) -> (w372:i32)
          n156 = Split 1D Array(array=w379, index=w380) -> (first subarray=w378:dbl[], second subarray=w376:dbl[])
          n157 = Split 1D Array(array=w369, index=w372) -> (first subarray=w370:dbl[], second subarray=w368:dbl[])
          n158 = call "Format Sum of Asymmetric Gaussians Fit Parameters.vi"("Step Size"=w366, "R^2"=w366, "MSE"=w366, "Best Fit Parameters"=w378) -> ("Array of Asymmetric Gaussian Fit Parameters"=w377:T13[])  [unwired: 6 in, 1 out]
          n159 = Index Array(array=w376) -> (element=w375:dbl)  [unwired: 1 in]
          n160 = call "Format Sum of Asymmetric Gaussians Fit Parameters.vi"("Step Size"=w384, "R^2"=w365, "MSE"=w385, "Best Fit Parameters"=w370) -> ("Array of Asymmetric Gaussian Fit Parameters"=w374:T13[])  [unwired: 6 in, 1 out]
          n161 = Index Array(array=w368) -> (element=w367:dbl)  [unwired: 1 in]
          n162 = Bundle(cluster=w373, "Asymmetric Gaussian Parameters"=w377, "Bridge Amplitude"=w375) -> (w382:T20)
          n163 = Bundle(cluster=w373, "Asymmetric Gaussian Parameters"=w374, "Bridge Amplitude"=w367) -> (w383:T20)
        }
        frame "Two T-Connected Asymmetric Gaussians" {
          w424 = T21 {"Asymmetric Gaussian Parameters"=[], "Bridge Amplitude"=0.0, "Bridge Slope"=0.0} ("Two T-Connected Asymmetric Gaussian Parameters")
          w422 = 0.0 ("MSE")
          n164 = Variant To Data(type=T5 {"Fix D-only Peak Location"=FALSE, "Peak Location"=0.0, "Fix D-only Peak FWHM"=FALSE, "Peak FWHM"=0.0} ("Fixed Parameters"), Variant=w454) -> (data=w453:T5)  [unwired: 1 in, 1 out]
          n165 = Unbundle By Name(w453) -> ("Fix D-only Peak FWHM"=w445:bool, "Peak FWHM"=w449:dbl, "Fix D-only Peak Location"=w447:bool, "Peak Location"=w450:dbl)
          n166 = case shown="True" w447 {
            tunnel: w452 -> [w476 w480]
            tunnel: [w476 w479] -> w451
            tunnel: w450 -> [_ w477]
            frame False {
            }
            frame True {
              n167 = Insert Into Array(array=w480, index=1 ("length"), new element=w477) -> (w479:dbl[])
            }
          }
          n168 = case shown="True" w445 {
            tunnel: w451 -> [w466 w471]
            tunnel: [w466 w475] -> w429
            tunnel: w449 -> [_ w473]
            frame False {
            }
            frame True {
              n169 = Index Array(array=w471, index=2) -> (element=w468:dbl)
              n170 = Absolute Value(x=w468) -> (abs(x)=w467:dbl)
              n171 = expression code="x/sqrt(2*ln(2))"(w473) -> (w472:dbl)
              n172 = Compound Arithmetic op=ADD(invert w467, w472) -> (w469:dbl)
              n173 = Insert Into Array(array=w471, index=3, new element=w469) -> (w475:dbl[])
            }
          }
          n174 = case shown="True" w447 {
            tunnel: w448 -> [w461 w465]
            tunnel: [w461 w464] -> w446
            frame False {
            }
            frame True {
              n175 = Insert Into Array(array=w465, index=1 ("length"), new element=0.0 ("new element/subarray")) -> (w464:dbl[])
            }
          }
          n176 = case shown="True" w445 {
            tunnel: w446 -> [w456 w460]
            tunnel: [w456 w459] -> w438
            frame False {
            }
            frame True {
              n177 = Insert Into Array(array=w460, index=3, new element=0.0 ("new element/subarray")) -> (w459:dbl[])
            }
          }
          n178 = Array Size(array=w438) -> (size(s)=w440:i32)
          n179 = Array Size(array=w429) -> (size(s)=w431:i32)
          n180 = expression code="x-2"(w440) -> (w439:i32)
          n181 = expression code="x-2"(w431) -> (w432:i32)
          n182 = Split 1D Array(array=w438, index=w439) -> (first subarray=w437:dbl[], second subarray=w435:dbl[])
          n183 = Split 1D Array(array=w429, index=w432) -> (first subarray=w430:dbl[], second subarray=w428:dbl[])
          n184 = call "Format Sum of Asymmetric Gaussians Fit Parameters.vi"("Step Size"=w422, "R^2"=w422, "MSE"=w422, "Best Fit Parameters"=w437) -> ("Array of Asymmetric Gaussian Fit Parameters"=w436:T13[])  [unwired: 6 in, 1 out]
          n185 = Index Array(array=w435) -> (element #1=w434:dbl, element #2=w426:dbl)  [unwired: 2 in]
          n186 = call "Format Sum of Asymmetric Gaussians Fit Parameters.vi"("Step Size"=w443, "R^2"=w423, "MSE"=w444, "Best Fit Parameters"=w430) -> ("Array of Asymmetric Gaussian Fit Parameters"=w433:T13[])  [unwired: 6 in, 1 out]
          n187 = Index Array(array=w428) -> (element #1=w427:dbl, element #2=w425:dbl)  [unwired: 2 in]
          n188 = Bundle By Name(cluster=w424, "Asymmetric Gaussian Parameters"=w436, "Bridge Amplitude"=w434, "Bridge Slope"=w426) -> (w441:T21)
          n189 = Bundle By Name(cluster=w424, "Asymmetric Gaussian Parameters"=w433, "Bridge Amplitude"=w427, "Bridge Slope"=w425) -> (w442:T21)
        }
        frame "1-Exponential" {
          w500 = T22 {"Amplitude"=0.0, "Time Constant"=0.0, "Baseline"=0.0, "Mean"=0.0, "SDV"=0.0, "FWHM"=0.0, "Integral"=0.0, "MSE"=0.0, "R^2"=0.0} ("Single Exponential Fit Parameters")
          n190 = Index Array(array=w496) -> (element #1=w491:dbl, element #2=w494:dbl, element #3=w485:dbl)  [unwired: 3 in]
          n191 = Index Array(array=w499) -> (element #1=w498:dbl, element #2=w497:dbl, element #3=w487:dbl)  [unwired: 3 in]
          n192 = Compound Arithmetic op=MULTIPLY(w491, w494, invert w483) -> (w490:dbl)
          n193 = Multiply(x=w483, y=w482) -> (x*y=w481:dbl)
          n194 = Compound Arithmetic op=ADD(w490, w481) -> (w484:dbl)
          n195 = Multiply(x=w494, y=0.6931471805599453) -> (x*y=w493:dbl)
          n196 = Bundle By Name(cluster=w500, "Amplitude"=w498, "Time Constant"=w497, "Baseline"=w487) -> (w489:T22)
          n197 = Bundle By Name(cluster=w500, "Amplitude"=w491, "Time Constant"=w494, "Baseline"=w485, "FWHM"=w493, "Integral"=w484, "MSE"=w492, "R^2"=w486) -> (w488:T22)
        }
        frame "Power Law with Offset" {
          w516 = T23 {"A"=0.0, "beta"=0.0, "B"=0.0, "Mean"=0.0, "SDV"=0.0, "Integral"=0.0, "MSE"=0.0, "R^2"=0.0} ("Power Law Fit Parameters")
          n198 = Index Array(array=w512) -> (element #1=w506:dbl, element #2=w505:dbl, element #3=w504:dbl)  [unwired: 3 in]
          n199 = Index Array(array=w515) -> (element #1=w514:dbl, element #2=w513:dbl, element #3=w508:dbl)  [unwired: 3 in]
          n200 = formula code="float64 xpo;\nxpo = 1 + beta;\nIGL = B*(xmax-xmin)+A/xpo*(xmax**xpo - xmin**xpo);"("A"=w506, "beta"=w505, "B"=w504, "xmin"=w502, "xmax"=w501) -> ("IGL"=w503:dbl)
          n201 = Bundle By Name(cluster=w516, "A"=w506, "beta"=w505, "B"=w504, "Integral"=w503, "MSE"=w511, "R^2"=w507) -> (w509:T23)
          n202 = Bundle By Name(cluster=w516, "A"=w514, "beta"=w513, "B"=w508) -> (w510:T23)
        }
        frame "Power Law" {
          w530 = T23 {"A"=0.0, "beta"=0.0, "B"=0.0, "Mean"=0.0, "SDV"=0.0, "Integral"=0.0, "MSE"=0.0, "R^2"=0.0} ("Power Law Fit Parameters")
          n203 = Index Array(array=w526) -> (element #1=w521:dbl, element #2=w520:dbl)  [unwired: 2 in]
          n204 = Index Array(array=w529) -> (element #1=w528:dbl, element #2=w527:dbl)  [unwired: 2 in]
          n205 = formula code="float64 xpo;\nxpo = 1 + beta;\nIGL = A/xpo*(xmax**xpo - xmin**xpo);"("A"=w521, "beta"=w520, "xmin"=w518, "xmax"=w517) -> ("IGL"=w519:dbl)
          n206 = Bundle By Name(cluster=w530, "A"=w521, "beta"=w520, "Integral"=w519, "MSE"=w525, "R^2"=w522) -> (w523:T23)
          n207 = Bundle By Name(cluster=w530, "A"=w528, "beta"=w527) -> (w524:T23)
        }
        frame "IRF*PSED" {
          w542 = nan ("FWHM")
          w559 = T24 {"Offset"=0.0, "Amplitudes"=[], "Time Constants"=[], "Baseline"=0.0, "Lifetime"=0.0, "IRF order"=0.0, "Period"=0.0, "SDV"=0.0, "FWHM"=0.0, "Integral"=0.0, "MSE"=0.0, "R^2"=0.0} ("IRF*PSED Fit Parameters")
          # "#TODO"
          n208 = Delete From Array(array=w552) -> (deleted portion=w551:dbl, array with subset deleted=w550:dbl[])  [unwired: 2 in]
          n209 = Delete From Array(array=w547) -> (deleted portion=w546:dbl, array with subset deleted=w544:dbl[])  [unwired: 2 in]
          n210 = Variant To Data(type=T6 {"order"=0, "T"=0.0, "Time Constant Array"=[], "{S_k, C_k, phi_k, e_k} arrays"={"S_k Array"=[], "C_k Array"=[], "phi_k Array"=[], "e_k Array"=[]}, "IRF Extraction Options"={"Time Constant for IRF Extraction"=1e-18, "IRF Order"=0, "Fourier Series Smoothing"=enum."None", "Noise Threshold"=0.0, "Smoothing Width"=0.0, "Fourier Series Truncation"=enum."Automatic", "Truncation Order"=0, "Save Power Spectrum"=FALSE, "Smoothing"=FALSE, "Smoothing Parameter"=0.0, "Smoothing Order"=1, "Method"=enum."Direct"}} ("IRF*PSED fixed Parameters"), Variant=w541) -> (data=w539:T6)  [unwired: 1 in, 1 out]
          n211 = Unbundle By Name(w539) -> ("IRF Extraction Options.Time Constant for IRF Extraction"=w538:dbl[unit], "T"=w537:dbl, "Time Constant Array"=w534:dbl[])
          n212 = Multiply(x=w554, y=w553) -> ()  [unwired: 1 out]
          n213 = Delete From Array(array=w550, index=0) -> (deleted portion=w548:dbl, array with subset deleted=w536:dbl[])  [unwired: 1 in]
          n214 = Delete From Array(array=w544, index=0) -> (deleted portion=w543:dbl, array with subset deleted=w535:dbl[])  [unwired: 1 in]
          n215 = Increment(x=w532) -> (x+1=w531:i32)
          n216 = node(w538) -> (w533:dbl)
          n217 = Bundle By Name(cluster=w559, "Lifetime"=w533, "IRF order"=w531, "Period"=w537, "Offset"=w543, "Amplitudes"=w535, "Time Constants"=w534, "Baseline"=w546, "FWHM"=w542, "Integral"=w542, "MSE"=w558, "R^2"=w555) -> (w556:T24)
          n218 = Bundle By Name(cluster=w559, "Offset"=w548, "Amplitudes"=w536, "Baseline"=w551) -> (w557:T24)
        }
        frame "2-Exponentials" {
          w569 = T25 {"A1"=0.0, "tau1"=0.0, "A2"=0.0, "tau2"=0.0, "Baseline"=0.0, "Mean"=0.0, "SDV"=0.0, "Integral"=0.0, "MSE"=0.0, "R^2"=0.0} ("Double Exponential Fit Parameters")
          n219 = Index Array(array=w575) -> (element #1=w567:dbl, element #2=w566:dbl, element #3=w565:dbl, element #4=w564:dbl, element #5=w560:dbl)  [unwired: 5 in]
          n220 = formula code="float64 N;\nN = A1*t1+A2*t2;\nm = (A1*t1**2+A2*t2**2)/N;\ns = 2*sqrt(A1*t1*A2*t2)*abs(t2-t1)/N;\nI = (A1*t1 + A2*t2)/dt;"("t1"=w566, "A2"=w565, "t2"=w564, "dt"=w574, "A1"=w567, "nb"=w561, "B"=w560) -> ("m"=w573:dbl, "s"=w572:dbl, "I"=w571:dbl)
          n221 = Index Array(array=w581) -> (element #1=w580:dbl, element #2=w579:dbl, element #3=w578:dbl, element #4=w577:dbl, element #5=w562:dbl)  [unwired: 5 in]
          n222 = Bundle By Name(cluster=w569, "A1"=w580, "tau1"=w579, "A2"=w578, "tau2"=w577, "Baseline"=w562) -> (w576:T25)
          n223 = Bundle By Name(cluster=w569, "A1"=w567, "tau1"=w566, "A2"=w565, "tau2"=w564, "Baseline"=w560, "Mean"=w573, "SDV"=w572, "MSE"=w570, "Integral"=w571, "R^2"=w563) -> (w568:T25)
        }
        frame "2D Gaussian ACF" {
          w592 = T26 {"Amplitude"=0.0, "Diffusion Time"=0.0, "RMSE"=0.0, "R^2"=0.0} ("2D ACF Fit Parameters")
          n224 = Index Array(array=w587) -> (element #1=w586:dbl, element #2=w584:dbl)  [unwired: 2 in]
          n225 = Index Array(array=w590) -> (element #1=w583:dbl, element #2=w582:dbl)  [unwired: 2 in]
          n226 = Bundle By Name(cluster=w592, "Amplitude"=w586, "Diffusion Time"=w584) -> (w589:T26)
          n227 = Bundle By Name(cluster=w592, "Amplitude"=w583, "Diffusion Time"=w582, "RMSE"=w591, "R^2"=w585) -> (w588:T26)
        }
        frame "2D Gaussian + Blinking ACF" {
          w607 = T27 {"Amplitude"=0.0, "Diffusion Time"=0.0, "Blinking Fraction"=0.0, "Blinking Time Constant"=0.0, "RMSE"=0.0, "R^2"=0.0} ("2D Gaussian + Blinking ACF Fit Parameters")
          n228 = Index Array(array=w605) -> (element #1=w598:dbl, element #2=w597:dbl, element #3=w594:dbl, element #4=w593:dbl)  [unwired: 4 in]
          n229 = Index Array(array=w602) -> (element #1=w601:dbl, element #2=w599:dbl, element #3=w596:dbl, element #4=w595:dbl)  [unwired: 4 in]
          n230 = Bundle By Name(cluster=w607, "Amplitude"=w601, "Diffusion Time"=w599, "Blinking Fraction"=w596, "Blinking Time Constant"=w595) -> (w604:T27)
          n231 = Bundle By Name(cluster=w607, "Amplitude"=w598, "Diffusion Time"=w597, "Blinking Fraction"=w594, "Blinking Time Constant"=w593, "RMSE"=w606, "R^2"=w600) -> (w603:T27)
        }
        frame "2D Gaussian + Flow ACF" {
          w620 = T28 {"Amplitude"=0.0, "Diffusion Time"=0.0, "Translation Time"=0.0, "RMSE"=0.0, "R^2"=0.0} ("2D Gaussian + Blinking ACF Fit Parameters")
          n232 = Index Array(array=w618) -> (element #1=w611:dbl, element #2=w610:dbl, element #3=w608:dbl)  [unwired: 3 in]
          n233 = Index Array(array=w615) -> (element #1=w614:dbl, element #2=w612:dbl, element #3=w609:dbl)  [unwired: 3 in]
          n234 = Bundle By Name(cluster=w620, "Amplitude"=w614, "Diffusion Time"=w612, "Translation Time"=w609) -> (w617:T28)
          n235 = Bundle By Name(cluster=w620, "Amplitude"=w611, "Diffusion Time"=w610, "Translation Time"=w608, "RMSE"=w619, "R^2"=w613) -> (w616:T28)
        }
        frame "3D Gaussian ACF" {
          w625 = T29 {"Amplitude"=0.0, "Diffusion Time"=0.0, "Aspect Ratio"=0.0, "RMSE"=0.0, "R^2"=0.0} ("3D ACF Fit Parameters")
          n236 = Index Array(array=w630) -> (element #1=w623:dbl, element #2=w628:dbl, element #3=w624:dbl)  [unwired: 3 in]
          n237 = Index Array(array=w633) -> (element #1=w627:dbl, element #2=w626:dbl, element #3=w622:dbl)  [unwired: 3 in]
          n238 = Absolute Value(x=w622) -> (abs(x)=w621:dbl)
          n239 = Bundle By Name(cluster=w625, "Amplitude"=w623, "Diffusion Time"=w628, "Aspect Ratio"=w624) -> (w632:T29)
          n240 = Bundle By Name(cluster=w625, "Amplitude"=w627, "Diffusion Time"=w626, "Aspect Ratio"=w621, "RMSE"=w634, "R^2"=w629) -> (w631:T29)
        }
        frame "3D Gaussian + Blinking ACF" {
          w641 = T30 {"Amplitude"=0.0, "Diffusion Time"=0.0, "Aspect Ratio"=0.0, "Blinking Fraction"=0.0, "Blinking Time Constant"=0.0, "RMSE"=0.0, "R^2"=0.0} ("2D Gaussian + Blinking ACF Fit Parameters")
          n241 = Index Array(array=w650) -> (element #1=w643:dbl, element #2=w642:dbl, element #3=w635:dbl, element #4=w636:dbl, element #5=w637:dbl)  [unwired: 5 in]
          n242 = Index Array(array=w647) -> (element #1=w646:dbl, element #2=w644:dbl, element #3=w638:dbl, element #4=w639:dbl, element #5=w640:dbl)  [unwired: 5 in]
          n243 = Bundle By Name(cluster=w641, "Amplitude"=w643, "Diffusion Time"=w642, "Aspect Ratio"=w635, "Blinking Fraction"=w636, "Blinking Time Constant"=w637, "RMSE"=w651, "R^2"=w645) -> (w648:T30)
          n244 = Bundle By Name(cluster=w641, "Amplitude"=w646, "Diffusion Time"=w644, "Aspect Ratio"=w638, "Blinking Fraction"=w639, "Blinking Time Constant"=w640) -> (w649:T30)
        }
        frame "2D Gaussian ACF & 2D Gaussian + Flow ACF" {
          w654 = T31 {"Amplitude 1"=0.0, "Diffusion Time"=0.0, "Amplitude 2"=0.0, "Translation Time"=0.0, "RMSE"=0.0, "R^2"=0.0} ("2D Gaussian ACF & ACF + Flow Fit Parameters")
          n245 = Index Array(array=w662) -> (element #1=w661:dbl, element #2=w659:dbl, element #3=w653:dbl, element #4=w656:dbl)  [unwired: 4 in]
          n246 = Index Array(array=w665) -> (element #1=w658:dbl, element #2=w657:dbl, element #3=w652:dbl, element #4=w655:dbl)  [unwired: 4 in]
          n247 = Bundle By Name(cluster=w654, "Amplitude 1"=w661, "Diffusion Time"=w659, "Amplitude 2"=w653, "Translation Time"=w656) -> (w664:T31)
          n248 = Bundle By Name(cluster=w654, "Amplitude 1"=w658, "Diffusion Time"=w657, "Amplitude 2"=w652, "Translation Time"=w655, "RMSE"=w666, "R^2"=w660) -> (w663:T31)
        }
      }
    }
    frame Error {
    }
  }
  "Fit Parameters Cluster" <- w8
  "Fit Parameters Uncertainties Cluster" <- w9
  "Error Out" <- w2
